vi "Three 8-bit Port Digital Input.vi"(2 "Three 8-bit DI Ports":T1={"8-bit DI Port 0"="Chassis1/Mod4/DI7:0", "8-bit DI Port 1"="Chassis1/Mod4/DI7:0", "8-bit DI Port 2"="Chassis1/Mod4/DI7:0"}) -> (7 "Packet":u64)   [LabVIEW 2009]
uses:
  <vilib>/eio/EIONode/EIONode.xnode
  <vilib>/rvi/eio/nirviEIOImplementation/nirviEIOImplementation.xnode
  <vilib>/rvi/eio/common/nirviEmuTemplateMethod_noerrors.vi
  <vilib>/rvi/eio/common/nirviEmuClasses.ctl
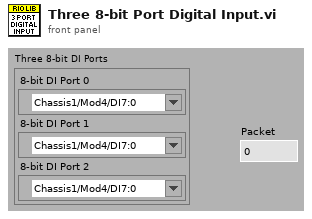
[diagram p1: front panel]
types:
  T1 = cluster{"8-bit DI Port 0":refnum<k21>, "8-bit DI Port 1":refnum<k21>, "8-bit DI Port 2":refnum<k21>}
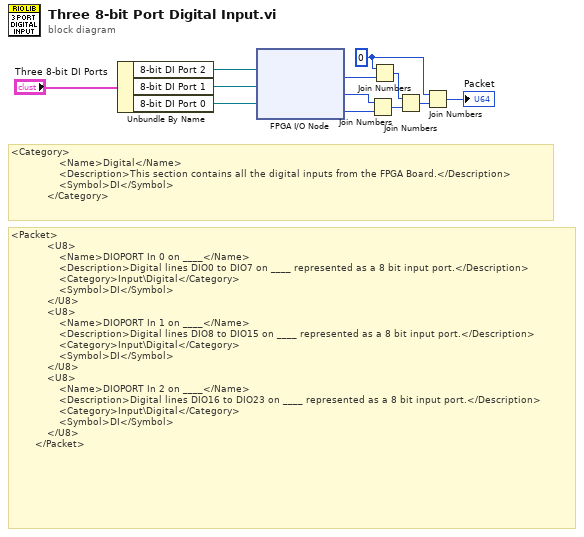
[diagram p0: block diagram]
diagram:
  w2 = u8 0 ("hi")
  # "<Packet>\n            <U8>\n                <Name>DIOPORT In 0 on ____</Name>\n                <Description>Digital lines DIO0 to DIO7 on ____ represented as a 8 bit input port.</Description>\n                <Category>Input\\Digital</Category>\n                <Symbol>DI</Symbol>\n            </U8>\n            <U8>\n                <Name>DIOPORT In 1 on ____</Name>\n                <Description>Digital lines DIO8 to DIO15 on ____ represented as a 8 bit input port.</Description>\n                <Category>Input\\Digital</Category>\n                <Symbol>DI</Symbol>\n            </U8>\n            <U8>\n                <Name>DIOPORT In 2 on ____</Name>\n                <Description>Digital lines DIO16 to DIO23 on ____ represented as a 8 bit input port.</Description>\n                <Category>Input\\Digital</Category>\n                <Symbol>DI</Symbol>\n            </U8>\n        </Packet>"
  # "<Category>\n                <Name>Digital</Name>\n                <Description>This section contains all the digital inputs from the FPGA Board.</Description>\n                <Symbol>DI</Symbol>\n            </Category>"
  n1 = Unbundle By Name("Three 8-bit DI Ports") -> ("8-bit DI Port 2"=w5:refnum<k21>, "8-bit DI Port 1"=w7:refnum<k21>, "8-bit DI Port 0"=w8:refnum<k21>)
  n2 = xnode "FPGA I/O Node"("FPGA I/O In"=w5, "FPGA I/O In"=w7, "FPGA I/O In"=w8) -> ("I/O Item"=w3:u8, "I/O Item"=w6:u8, "I/O Item"=w11:u8)  [unwired: 3 out]
  n3 = Join Numbers(hi=w6, lo=w11) -> ((hi.lo)=w4:u16)
  n4 = Join Numbers(hi=w2, lo=w3) -> ((hi.lo)=w1:u16)
  n5 = Join Numbers(hi=w1, lo=w4) -> ((hi.lo)=w12:u32)
  n6 = Join Numbers(hi=w2, lo=w12) -> ((hi.lo)=→"Packet":u64)
